vi "Dummy Input.vi"(7 "error in (no error)":errorcluster) -> (0 "error out":errorcluster, 2 "Multi Input":dbl[](array[numeric]) format="%#.2g", 3 "Single Input":dbl format="%#.2g")   [LabVIEW 2023]
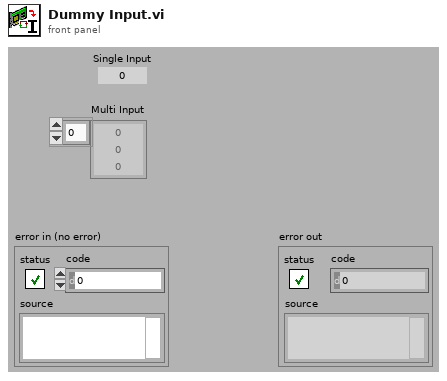
[diagram p1: front panel]
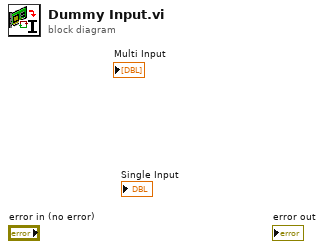
[diagram p0: block diagram]
diagram:
